vi "Initialize.vi"(8 "error in (no error)":errorcluster, 11 "Ismatech 3 Channel Settings In":T1 {"Channel Number" min=0 max=3; "Pump Number" min=1 max=9}) -> (0 "error out":errorcluster, 1 "Initialized":bool, 2 "No Pump Connected":bool=TRUE, 3 "Ismatech 3 Channel Settings Out":T1={"VISA resource name"="", "Pump Number"=1, "Channel Number"=0, "Simulated?"=TRUE, "Reverse?"=FALSE} {"Channel Number" min=0 max=3; "Pump Number" min=1 max=9}, 4 "1st Reserve":i32, 5 "2nd Reserved":i32, 6 "2nd Release":i32, 7 "Status Completed":bool)   [LabVIEW 2018, in "Ismatec 4308.lvlib"]
uses:
  Ismatec 4308.lvlib
  Ismatec 4083.ctl
  <vilib>/Instr/_visa.llb/VISA Configure Serial Port (Instr).vi
  support/Support Library.lvlib
panel:
  out "1st Release 2":i32
  out "1st Release":i32
  out "read buffer 4":string
  out "read buffer 3":string
  out "read buffer 2":string
  out "read buffer":string
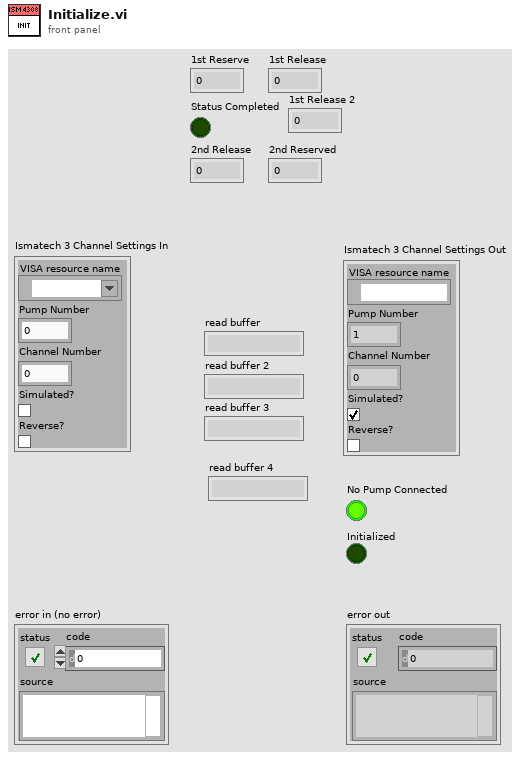
[diagram p1: front panel]
types:
  T1 = typedef "Ismatec 4308.lvlib/Ismatec 4083.ctl" = cluster{"VISA resource name":refnum<visa-resource-name>, "Pump Number":i16, "Channel Number":i16, "Simulated?":bool, "Reverse?":bool}
  T2 = typedef "Ismatec 4308.lvlib/Ismatec 4083 Global.ctl" = T3[]
  T3 = typedef "Ismatec 4308.lvlib/Ismatec 4083 Global Element.ctl" = cluster{"Busy":bool, "ChannelCnt":dbl, "Initialized":bool, "Current Channel":dbl, "Initialized Channels":dbl[]}
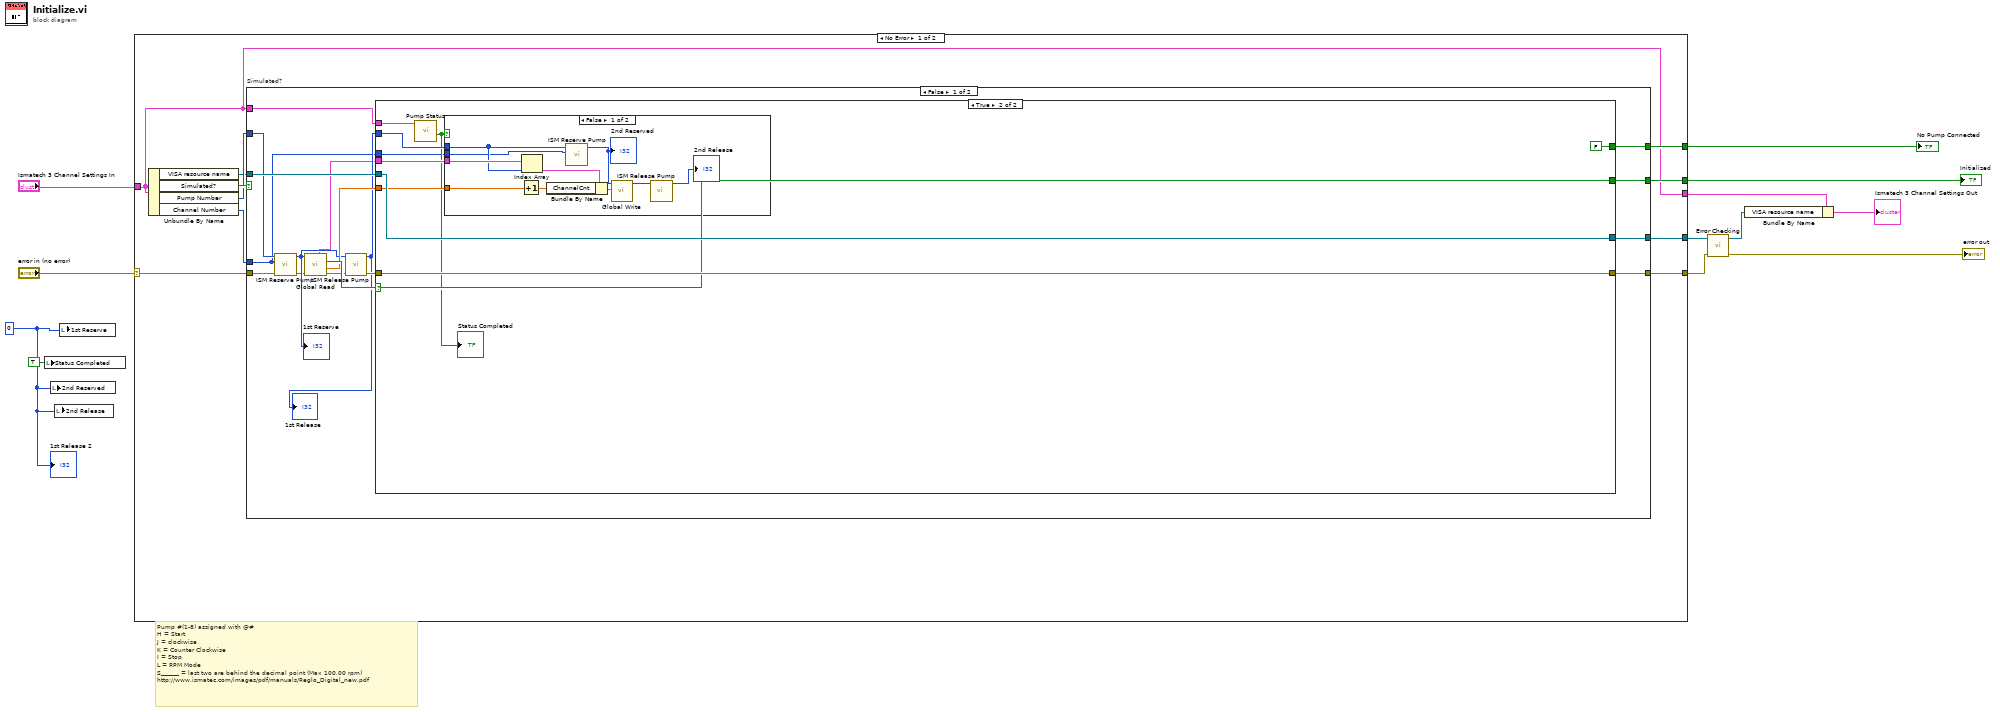
[diagram p0: block diagram]
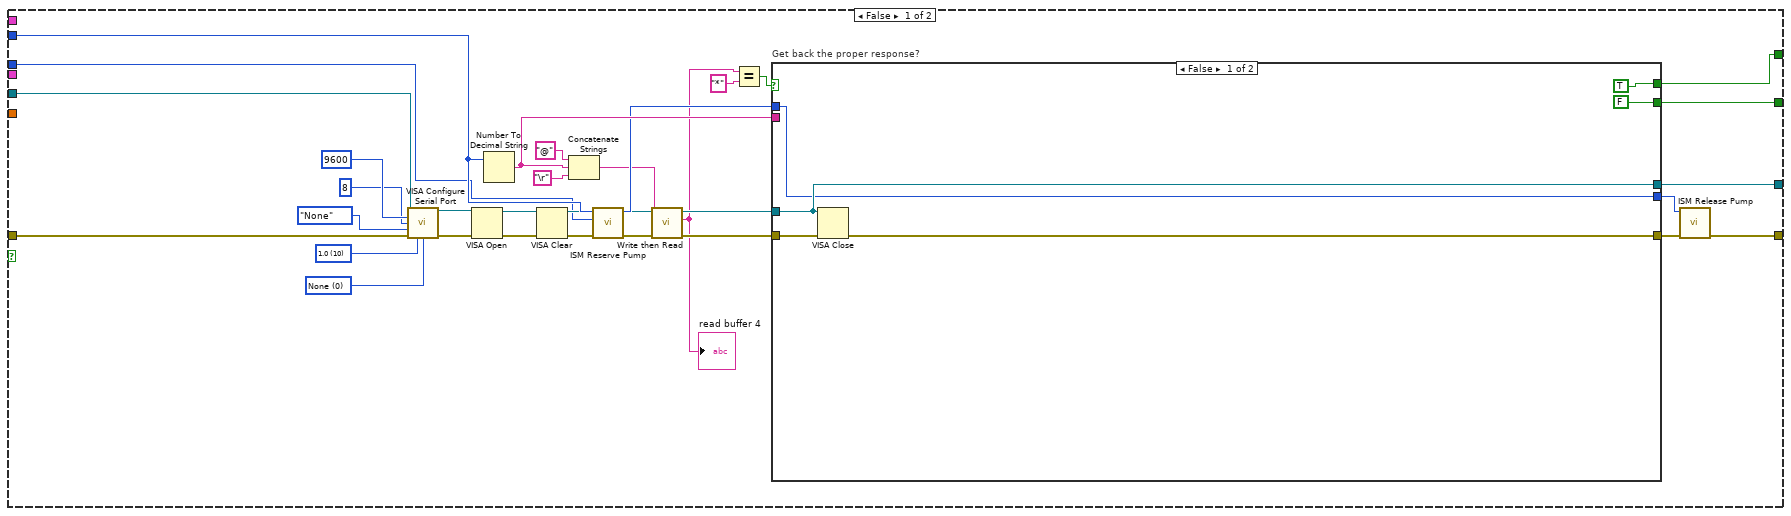
[diagram p2: hidden frame]
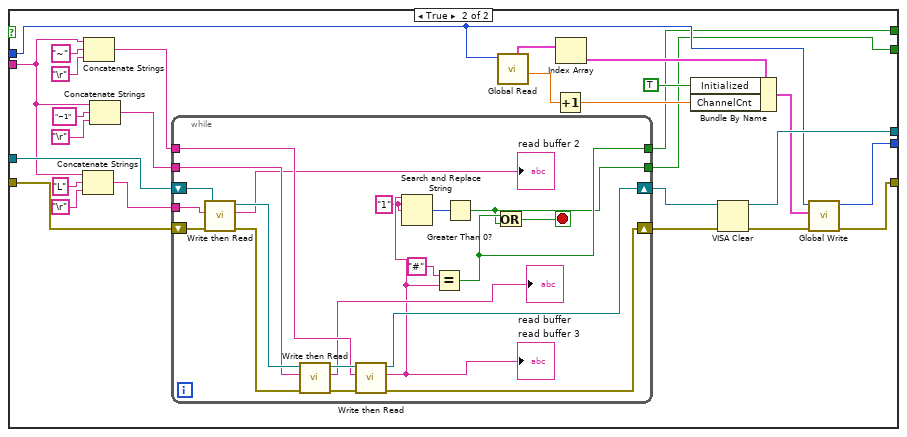
[diagram p3: hidden frame]
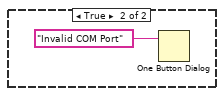
[diagram p4: hidden frame]
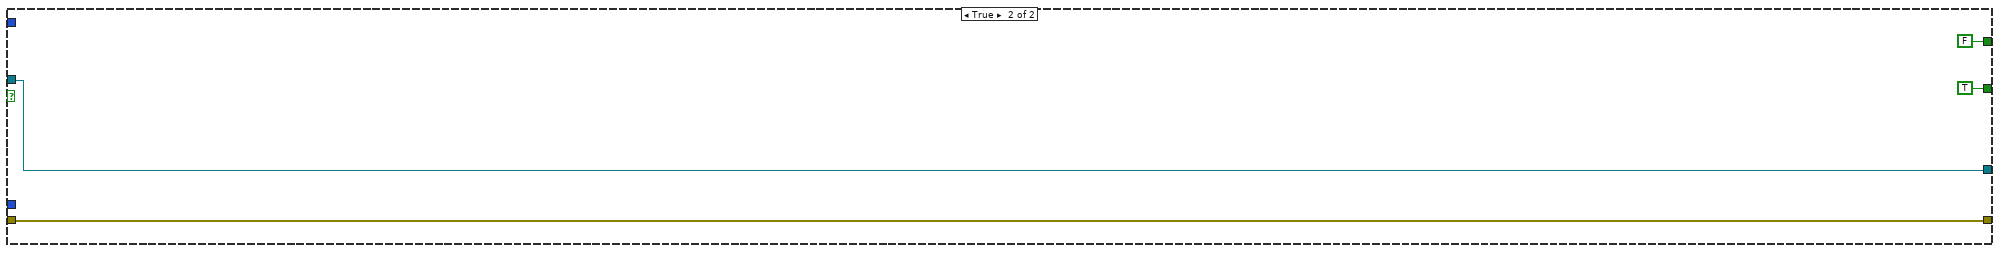
[diagram p5: hidden frame]
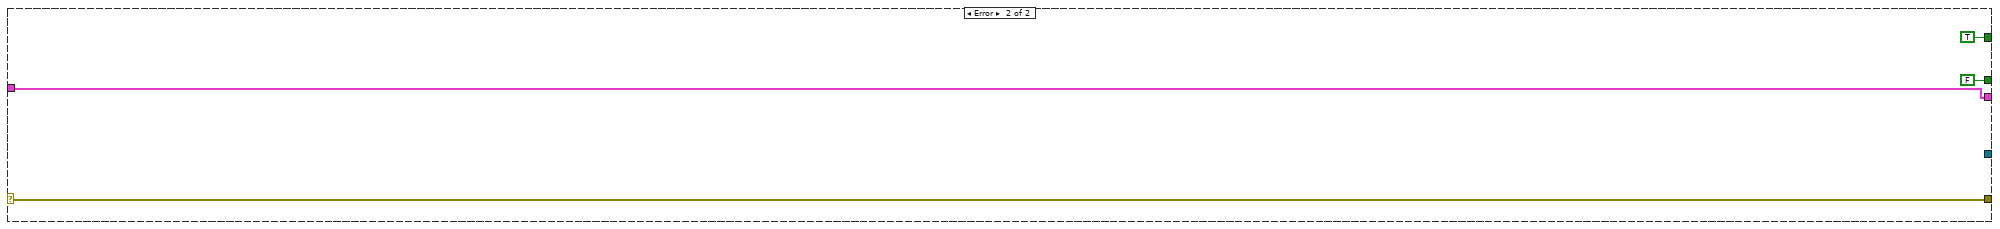
[diagram p6: hidden frame]
diagram:
  w1 = 0
  # "Pump #(1-8) assigned with @#\nH = Start\nJ = clockwise\nK = Counter Clockwise\nI = Stop\nL = RPM Mode\nS______ = last two are behind the decimal point (Max 100.00 rpm)\nhttp://www.ismatec.com/images/pdf/manuals/Reglo_Digital_new.pdf"
  n1 = local write "Status Completed"(TRUE ("Connection Error")) -> ()
  n2 = local write "2nd Reserved"(w1) -> ()
  n3 = local write "2nd Release"(w1) -> ()
  n4 = local write "1st Reserve"(w1) -> ()
  n5 = case shown="No Error" "error in (no error)" {
    selector: "error in (no error)" -> [w18 w153]
    tunnel: "Ismatech 3 Channel Settings In" -> [w14 w152]
    tunnel: [w21 w153] -> w9
    tunnel: [w14 w152] -> w8
    tunnel: [w17 _] -> w7
    tunnel: [w16 FALSE] -> w6
    tunnel: [w15 TRUE] -> w3
    frame No Error {
      n6 = Unbundle By Name(w14) -> ("VISA resource name"=w19:refnum<visa-resource-name>, "Simulated?"=w22:bool, "Pump Number"=w20:i16, "Channel Number"=w13:i16)
      n7 = case "Simulated?" shown="False" w22 {
        tunnel: [w36 w148] -> w21
        tunnel: [w37 w149] -> w17
        tunnel: w20 -> [w32 _]
        tunnel: w19 -> [w39 w149]
        tunnel: w18 -> [w27 w148]
        tunnel: [w38 TRUE] -> w16
        tunnel: [w33 FALSE] -> w15
        tunnel: w14 -> [w31 _]
        tunnel: w13 -> [w23 _]
        frame False {
          n8 = call "ISM Reserve Pump.vi"("error in (no error)"=w27, "ISM Channel # In"=w23, "ISM Pump # In"=w32) -> ("error out"=w28:errorcluster, "ISM Pump # Out"=w30:i32)  [unwired: 7 in]
          "1st Reserve" <- w30
          n9 = call "Global Read.vi"("error in (no error)"=w28, "Pump Number"=w30) -> ("error out"=w29:errorcluster, "ChannelCnt"=w34:dbl, "Initialized"=w35:bool, "Ismatec 4083 Global"=w24:T2)  [unwired: 3 in, 3 out]
          n10 = call "ISM Release Pump.vi"("error in (no error)"=w29, "Pump Number In"=w30) -> ("error out"=w26:errorcluster, "Pump Number Out"=w25:i32)  [unwired: 8 in]
          "1st Release" <- w25
          n11 = case shown="True" w35 {
            selector: w35 -> [_ w132]
            tunnel: w39 -> [w67 w134]
            tunnel: w26 -> [w66 w133]
            tunnel: [w65 w132] -> w38
            tunnel: [w64 w134] -> w37
            tunnel: [w63 w133] -> w36
            tunnel: w25 -> [w62 w128]
            tunnel: w24 -> [_ w131]
            tunnel: w34 -> [_ w130]
            tunnel: [w61 FALSE] -> w33
            tunnel: w31 -> [_ w127]
            tunnel: w23 -> [w40 w125]
            frame False {
              w51 = u16 0 items=["None", "XON/XOFF", "RTS/CTS", "XON/XOFF & RTS/CTS", "DTR/DSR", "XON/XOFF & DTR/DSR"] ("flow control (0:none)")
              w52 = u16 10 items=["1.0"=10, "1.5"=15, "2.0"=20] ("stop bits (10: 1 bit)")
              n12 = call-poly "VISA Configure Serial Port"("VISA resource name"=w67, "baud rate (9600)"=u32 9600, "data bits (8)"=u16 8, "parity (0:none)"=enum16{"None", "Odd", "Even", "Mark", "Space"}."None", "error in (no error)"=w66, "stop bits (10: 1 bit)"=w52, "flow control (0:none)"=w51) -> ("VISA resource name out"=w59:refnum<visa-resource-name>, "error out"=w58:errorcluster)  [unwired: 7 in]
              n13 = VISA Open(error in (no error)=w58, VISA resource name=w59) -> (VISA resource name=w50:refnum<visa-resource-name>, error out=w49:errorcluster)  [unwired: 3 in]
              n14 = Number To Decimal String(number=w62) -> (decimal integer string=w69:string)  [unwired: 1 in]
              n15 = VISA Clear(VISA resource name=w50, error in (no error)=w49) -> (VISA resource name out=w47:refnum<visa-resource-name>, error out=w48:errorcluster)
              n16 = Concatenate Strings("@" ("string"), w69, "\r") -> (w46:string)
              n17 = call "ISM Reserve Pump.vi"("error in (no error)"=w48, "ISM Channel # In"=w40, "ISM Pump # In"=w62) -> ("error out"=w45:errorcluster, "ISM Pump # Out"=w68:i32)  [unwired: 7 in]
              n18 = call "Write then Read.vi"("error in"=w45, "write buffer"=w46, "VISA resource name in"=w47) -> ("error out"=w70:errorcluster, "read buffer"=w60:string, "VISA resource name out"=w71:refnum<visa-resource-name>)  [unwired: 6 in]
              "read buffer 4" <- w60
              n19 = Equal?(x=w60, y="*") -> (x = y?=w43:bool)
              n20 = case "Get back the proper response?" shown="False" w43 {
                tunnel: w71 -> [w73 w104]
                tunnel: w70 -> [w77 w103]
                tunnel: [w76 w86] -> w41
                tunnel: [TRUE w80] -> w61
                tunnel: [FALSE w81] -> w65
                tunnel: [w73 w98] -> w64
                tunnel: w69 -> [_ w79]
                tunnel: [w72 w88] -> w42
                tunnel: w68 -> [w72 w90]
                frame False {
                  n21 = VISA Close(VISA resource name=w73, error in (no error)=w77) -> (error out=w76:errorcluster)
                }
                frame True {
                  n22 = Concatenate Strings(w79, "L" ("string"), "\r") -> (w100:string)
                  n23 = Concatenate Strings(w79, "~" ("string"), "\r") -> (w82:string)
                  n24 = Concatenate Strings(w79, "~1" ("string"), "\r") -> (w97:string)
                  n25 = while {
                    tunnel: w100 -> [w114]
                    tunnel: w97 -> [w113]
                    shift-right: [w119] -> w95
                    shift-left: w104 -> [w122]
                    shift-right: [w118] -> w96
                    shift-left: w103 -> [w115]
                    tunnel: w82 -> [w112]
                    tunnel: [w108] -> w81
                    tunnel: [w109] -> w80
                    stop <- w123 stop-if-true
                    w106 = "1" ("search string")
                    n26 = call "Write then Read.vi"("error in"=w115, "write buffer"=w114, "VISA resource name in"=w122) -> ("error out"=w116:errorcluster, "read buffer"=→"read buffer 2":string, "VISA resource name out"=w121:refnum<visa-resource-name>)  [unwired: 6 in]
                    n27 = call "Write then Read.vi"("error in"=w116, "write buffer"=w113, "VISA resource name in"=w121) -> ("error out"=w117:errorcluster, "read buffer"=→"read buffer":string, "VISA resource name out"=w120:refnum<visa-resource-name>)  [unwired: 6 in]
                    n28 = call "Write then Read.vi"("error in"=w117, "write buffer"=w112, "VISA resource name in"=w120) -> ("error out"=w118:errorcluster, "read buffer"=w107:string, "VISA resource name out"=w119:refnum<visa-resource-name>)  [unwired: 6 in]
                    "read buffer 3" <- w107
                    n29 = Search and Replace String(input string=w107, search string=w106, replace string=w106) -> (number of replacements=w105:i32)  [unwired: 5 in, 3 out]
                    n30 = Equal?(x="#", y=w107) -> (x = y?=w109:bool)
                    n31 = Greater Than 0?(x=w105) -> (x > 0?=w108:bool)
                    n32 = Or(x=w109, y=w108) -> (x .or. y?=w123:bool)
                  }
                  n33 = call "Global Read.vi"("Pump Number"=w90) -> ("ChannelCnt"=w94:dbl, "Ismatec 4083 Global"=w78:T2)  [unwired: 4 in, 5 out]
                  n34 = Increment(x=w94) -> (x+1=w91:dbl)
                  n35 = Index Array(array=w78) -> (element=w93:T3)  [unwired: 1 in]
                  n36 = Bundle By Name(cluster=w93, "Initialized"=TRUE, "ChannelCnt"=w91) -> (w89:T3)
                  n37 = VISA Clear(VISA resource name=w95, error in (no error)=w96) -> (VISA resource name out=w98:refnum<visa-resource-name>, error out=w87:errorcluster)
                  n38 = call "Global Write.vi"("error in (no error)"=w87, "Incoming Cluster"=w89, "Pump Number In"=w90) -> ("error out"=w86:errorcluster, "Pump Number Out"=w88:i32)  [unwired: 7 in]
                }
              }
              n39 = call "ISM Release Pump.vi"("error in (no error)"=w41, "Pump Number In"=w42) -> ("error out"=w63:errorcluster)  [unwired: 8 in, 1 out]
            }
            frame True {
              n40 = call "Pump Status.vi"("Ismatech 3 Channel Settings In"=w127) -> ("Connection Error"=w126:bool)  [unwired: 6 in, 4 out]
              "Status Completed" <- w126
              n41 = case shown="False" w126 {
                tunnel: w131 -> [w141 _]
                tunnel: w130 -> [w140 _]
                tunnel: w128 -> [w137 _]
                tunnel: w125 -> [w135 _]
                frame False {
                  n42 = Increment(x=w140) -> (x+1=w142:dbl)
                  n43 = Index Array(array=w141, index=w137) -> (element=w143:T3)
                  n44 = Bundle By Name(cluster=w143, "ChannelCnt"=w142) -> (w144:T3)
                  n45 = call "ISM Reserve Pump.vi"("ISM Channel # In"=w135, "ISM Pump # In"=w137) -> ("ISM Pump # Out"=w138:i32)  [unwired: 8 in, 1 out]
                  "2nd Reserved" <- w138
                  n46 = call "Global Write.vi"("Incoming Cluster"=w144, "Pump Number In"=w138) -> ("Pump Number Out"=w139:i32)  [unwired: 8 in, 1 out]
                  n47 = call "ISM Release Pump.vi"("Pump Number In"=w139) -> ("Pump Number Out"=→"2nd Release":i32)  [unwired: 9 in, 1 out]
                }
                frame True {
                  n48 = One Button Dialog(message="Invalid COM Port") -> ()  [unwired: 1 in, 1 out]
                }
              }
            }
          }
        }
        frame True {
        }
      }
    }
    frame Error {
    }
  }
  "Initialized" <- w6
  "No Pump Connected" <- w3
  n49 = call "Error Checking.vi"("error in (no error)"=w9, "VISA resource name"=w7) -> ("error out"=→"error out":errorcluster, "VISA resource name"=w11:refnum<visa-resource-name>)  [unwired: 7 in, 1 out]
  n50 = Bundle By Name(cluster=w8, "VISA resource name"=w11) -> (→"Ismatech 3 Channel Settings Out":T1)
  "1st Release 2" <- w1
